vi "Sub_NumberToColorScale.vi"(1 "Lower bound":dbl, 2 "Value":dbl, 3 "Upper bound":dbl) -> (0 "Resulting color":u32(colorbox))   [LabVIEW 2018]
panel:
  out "b":dbl
  out "a":dbl
  out "x+y":dbl
  out "coerced(x)":dbl
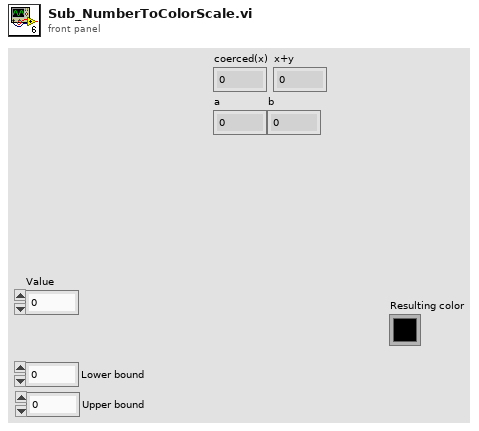
[diagram p1: front panel]
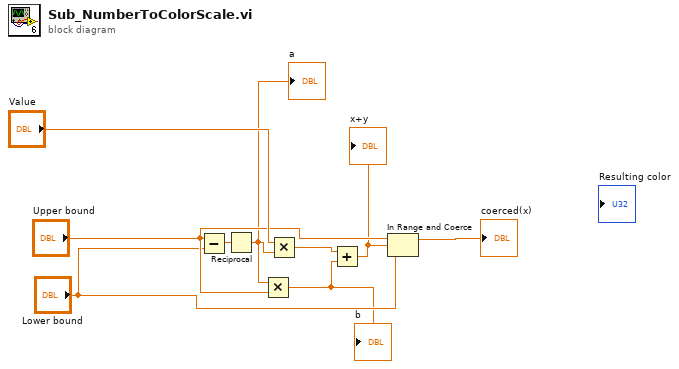
[diagram p0: block diagram]
diagram:
  n1 = Subtract(x="Upper bound", y="Lower bound") -> (x-y=w3:dbl)
  n2 = Reciprocal(x=w3) -> (1/x=w2:dbl)
  "a" <- w2
  n3 = Multiply(x=w2, y="Upper bound") -> (x*y=w1:dbl)
  "b" <- w1
  n4 = Multiply(x="Value", y=w2) -> (x*y=w8:dbl)
  n5 = Add(x=w8, y=w1) -> (x+y=w6:dbl)
  "x+y" <- w6
  n6 = In Range and Coerce(upper limit="Upper bound", x=w6, lower limit="Lower bound") -> (coerced(x)=→"coerced(x)":dbl)  [unwired: 1 out]
